vi "New Block UI.vi"(11 "Starting Name":string) -> (2 "Cancelled?":bool, 3 "New Block Config":T1={"Name"="", "Actions"={"Init"=FALSE, "Start"=FALSE, "Run"=TRUE, "Stop"=FALSE, "Close"=FALSE}, "IO Control"=FALSE, "New Project?"=FALSE, "Project"=refnum})   [LabVIEW 2022 SP3, in "FlexBlocks Support.lvlib"]
uses:
  FlexBlocks Support.lvlib
  Action Selections.ctl
  New Block Config.ctl
panel:
  in  "Enable IO Control":bool
  out "Action Diagram":picture
  out "Action Name":string
  out "Info":string
  in  "Actions":T2
  in  "Project Select":string(combo)
  in  "Add To Project":bool
  in  "Cancel":bool
  in  "OK":bool
  # "Enter the name of the new Worker to create:"
  # "Mouseover actions for descriptions."
  # "Unselected actions can later be added to workers by adding the specific case selection back in the Work.vi"
  # "Other Options"
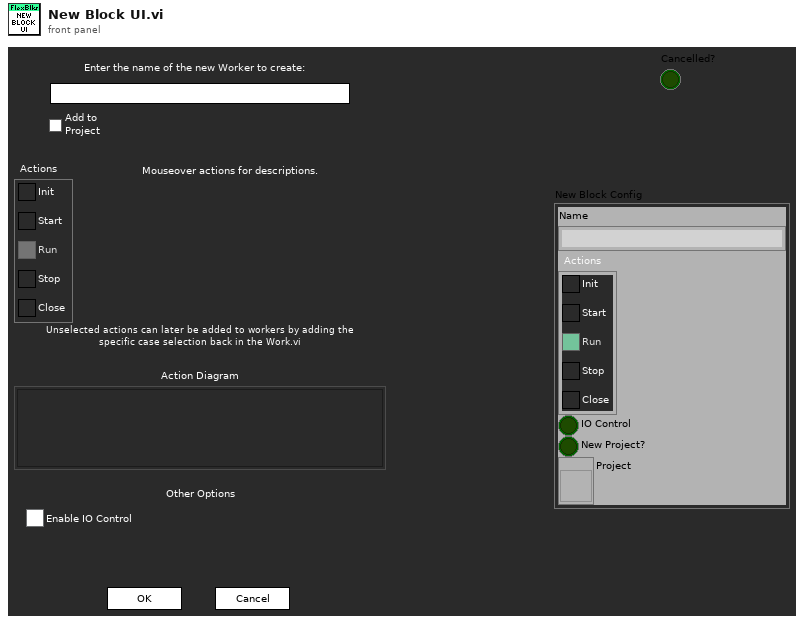
[diagram p1: front panel]
types:
  T1 = typedef "FlexBlocks Support.lvlib/New Block Config.ctl" = cluster{"Name":string, "Actions":T2, "IO Control":bool, "New Project?":bool, "Project":refnum<vi>}
  T2 = typedef "FlexBlocks Support.lvlib/Action Selections.ctl" = cluster{"Init":bool, "Start":bool, "Run":bool, "Stop":bool, "Close":bool}
  T3 = cluster{"Init":bool, "Start":bool, "Run":bool, "Stop":bool, "Close":bool}
  T4 = typedef "FlexBlocks Support.lvlib/Paths.ctl" = cluster{"FlexBlocks":path, "Workers Root":path, "Specialized Editors":path, "Worker Template":path, "SM Template":path, "Read Control Value Vim":path, "Write Indicator Value Vim":path, "XNode":path}
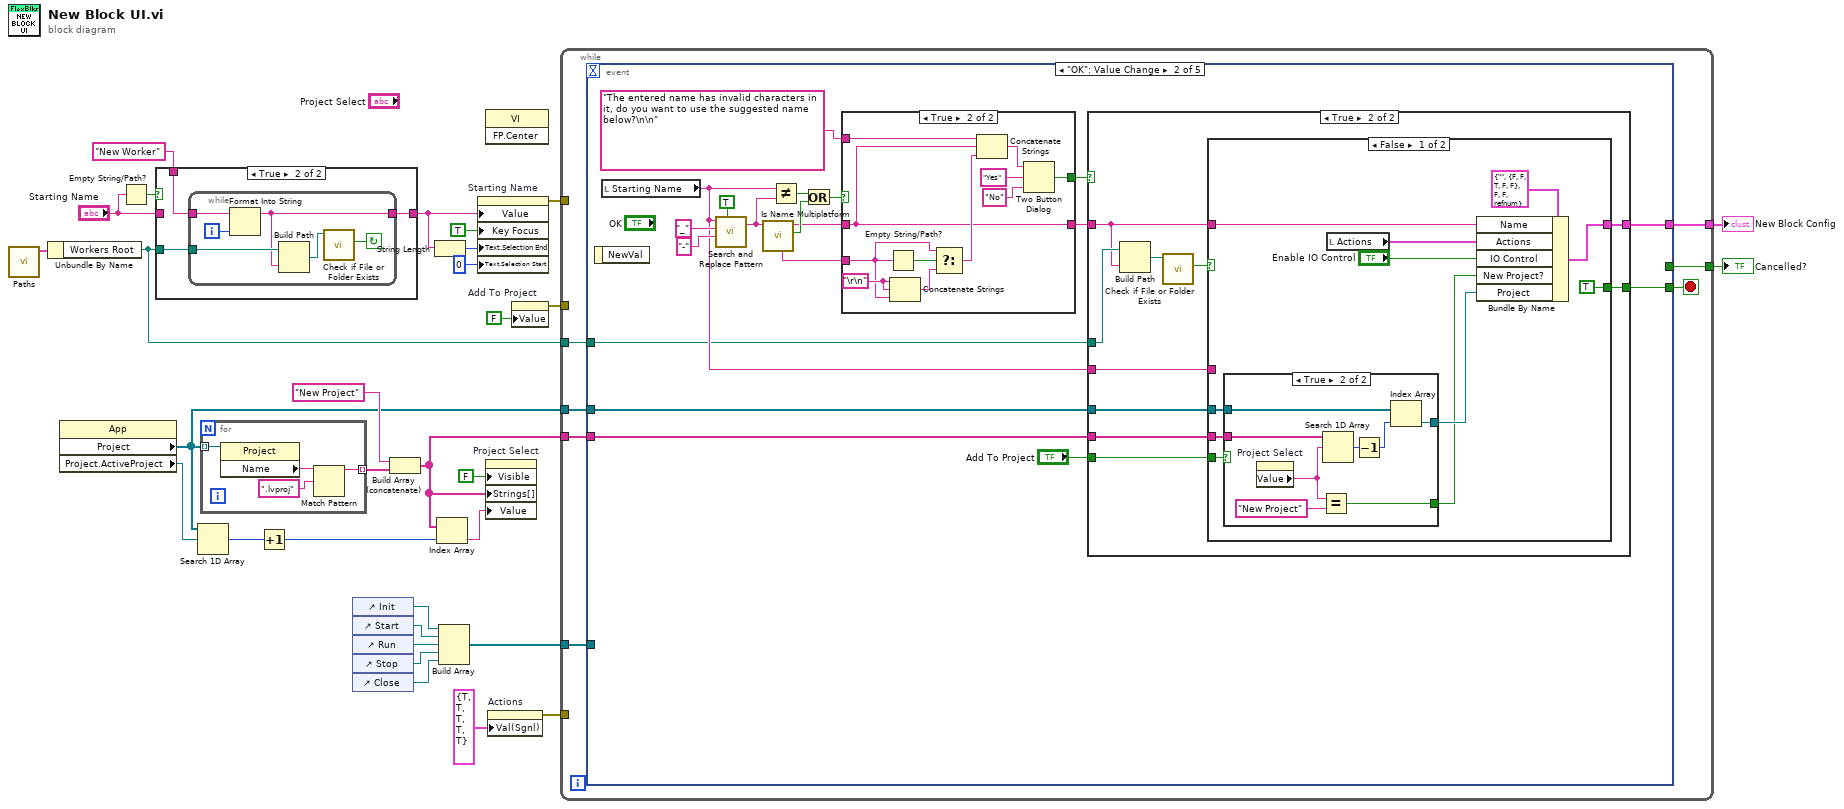
[diagram p0: block diagram]
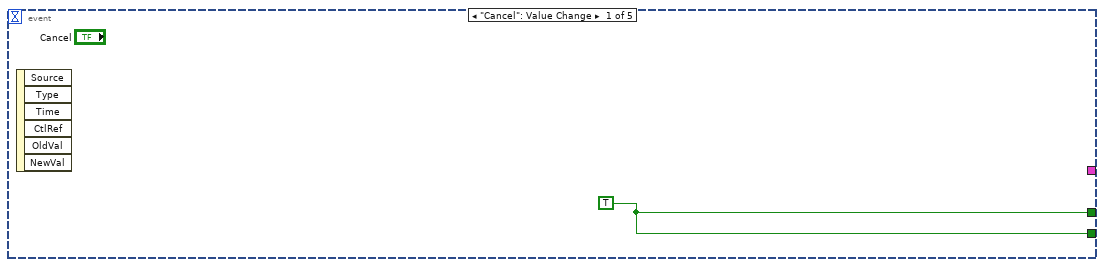
[diagram p2: hidden frame]
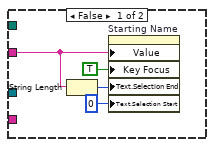
[diagram p3: hidden frame]
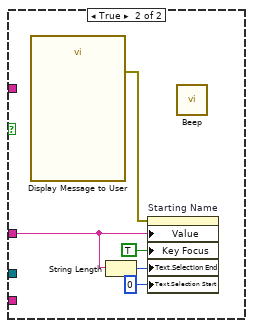
[diagram p5: hidden frame]
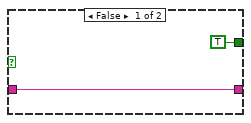
[diagram p6: hidden frame]
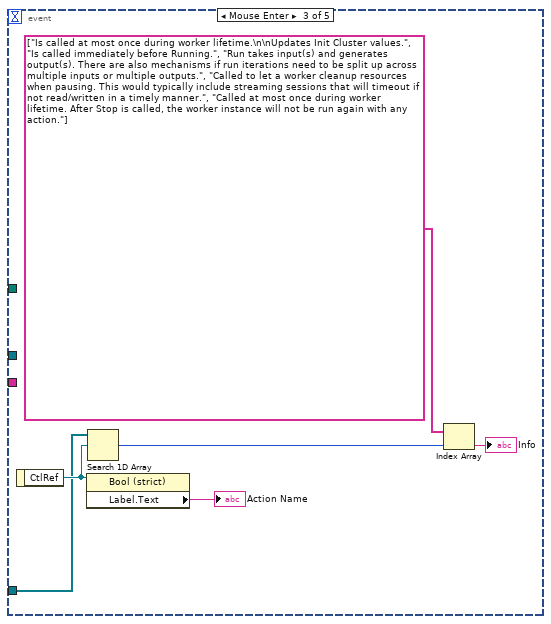
[diagram p7: hidden frame]
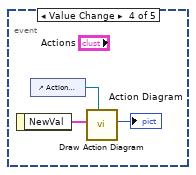
[diagram p8: hidden frame]
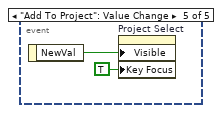
[diagram p9: hidden frame]
diagram:
  n1 = call "Paths.vi"() -> ("Paths"=w16:T4)  [unwired: 11 in]
  n2 = Unbundle By Name(w16) -> ("Workers Root"=w10:path)
  n3 = property class="App"() -> ("Project"=w13:refnum<vi>[], "Project.ActiveProject"=w22:refnum<vi>)  [unwired: 2 in, 2 out]
  n4 = Empty String/Path?(string/path="Starting Name") -> (empty?=w29:bool)
  n5 = case shown="True" w29 {
    tunnel: "Starting Name" -> [w32 _]
    tunnel: w10 -> [_ w35]
    tunnel: [w32 w34] -> w25
    tunnel: "New Worker" -> [_ w33]
    frame False {
    }
    frame True {
      n6 = while {
        tunnel: w35 -> [w40]
        tunnel: [w37] -> w34
        tunnel: w33 -> [w36]
        i -> [w41]
        stop <- w38 continue-if-true
        n7 = Format Into String(initial string=w36, w41) -> (resulting string=w37:string)  [unwired: 2 in, 1 out]
        n8 = Build Path(base path=w40, name or relative path=w37) -> (appended path=w39:path)
        n9 = call <vilib>:"Check if File or Folder Exists.vi"("path"=w39) -> ("file or folder exists?"=w38:bool)  [unwired: 8 in, 2 out]
      }
    }
  }
  n10 = Search 1D Array(1D array=w13, element=w22) -> (index of element=w21:i32)  [unwired: 1 in]
  n11 = for {
    tunnel: w13 -> [w45] mode=indexing
    tunnel: [w42] -> w19 mode=indexing
    n12 = property class="Project"(reference=w45) -> ("Name"=w44:string)  [unwired: 1 in, 2 out]
    n13 = Match Pattern(string=w44, regular expression=".lvproj") -> (before substring=w42:string)  [unwired: 1 in, 3 out]
  }
  n14 = Increment(x=w21) -> (x+1=w17:i32)
  n15 = control-ref of="Init"() -> (w5:refnum<vi>)
  n16 = control-ref of="Start"() -> (w6:refnum<vi>)
  n17 = control-ref of="Run"() -> (w9:refnum<vi>)
  n18 = control-ref of="Stop"() -> (w8:refnum<vi>)
  n19 = control-ref of="Close"() -> (w7:refnum<vi>)
  n20 = Build Array (concatenate)("New Project", w19) -> (w12:string[])
  n21 = String Length(string=w25) -> (length=w27:i32)
  n22 = Index Array(array=w12, index=w17) -> (element=w20:string)
  n23 = Build Array(w5, w6, w9, w8, w7) -> (w4:refnum<vi>[])
  n24 = property on="Starting Name" class="Str"("Value"=w25, "Key Focus"=TRUE, "Text.Selection End"=w27, "Text.Selection Start"=u32 0 ("Text.Selection:Start")) -> (error out=w15:errorcluster)  [unwired: 2 in, 1 out]
  n25 = invoke class="VI" method="FP.Center"() -> ()  [unwired: 3 in, 3 out]
  n26 = property on="Project Select" class="CmbBox"("Visible"=FALSE, "Strings[]"=w12, "Value"=w20) -> ()  [unwired: 2 in, 2 out]
  n27 = property on="Actions" class="Clust (strict)"("Val(Sgnl)"=T3 {"Init"=TRUE, "Start"=TRUE, "Run"=TRUE, "Stop"=TRUE, "Close"=TRUE} ("Value (Signaling)")) -> (error out=w3:errorcluster)  [unwired: 2 in, 1 out]
  n28 = property on="Add To Project" class="Bool (strict)"("Value"=FALSE ("Add To Project")) -> (error out=w14:errorcluster)  [unwired: 2 in, 1 out]
  n29 = while {
    tunnel: w15 -> [_]
    tunnel: w14 -> [_]
    tunnel: w13 -> [w50]
    tunnel: w12 -> [w49]
    tunnel: [w51] -> w11
    tunnel: [w48] -> w1
    tunnel: w10 -> [w47]
    tunnel: w4 -> [w46]
    tunnel: w3 -> [_]
    stop <- w52 stop-if-true
    n30 = event shown="[1] \"OK\": Value Change" {
      selector: _ -> [_ _ _ _ _]
      dyn-events: _ -> [_ _ _ _ _]
      timeout: _ -> [_ _ _ _ _]
      tunnel: [w53 w57 _ _ _] -> w52
      tunnel: [w53 _ _ _ _] -> w51
      tunnel: w50 -> [_ w59 _ _ _]
      tunnel: w49 -> [_ w58 _ _ _]
      tunnel: [_ w56 _ _ _] -> w48
      tunnel: w47 -> [_ w54 _ _ _]
      tunnel: w46 -> [_ _ w127 _ _]
      event "Cancel": Value Change {
        w53 = TRUE
        n31 = event-data() -> ()  [unwired: 1 in, 6 out]
      }
      event "OK": Value Change {
        n32 = event-data() -> ()  [unwired: 1 in, 1 out]
        n33 = local read "Starting Name"() -> (w55:string)
        n34 = call <vilib>:"Search and Replace Pattern.vi"("string"=w55, "regular expression (\"\")"="_" ("regular expression (\"\")"), "replace string (\"\")"="-" ("replace string (\"\")"), "replace all? (F)"=TRUE) -> ("result string"=w66:string)  [unwired: 1 in, 1 out]
        n35 = call <vilib>:"Is Name Multiplatform.vi"("filename"=w66) -> ("filename had conflict"=w71:bool, "suggested filename"=w70:string, "problem description"=w72:string)  [unwired: 6 in, 2 out]
        n36 = Not Equal?(x=w55, y=w66) -> (x != y?=w64:bool)
        n37 = Or(x=w64, y=w71) -> (x .or. y?=w65:bool)
        n38 = case shown="True" w65 {
          tunnel: w72 -> [_ w117]
          tunnel: w70 -> [w112 w113]
          tunnel: "The entered name has invalid characters in it, do you want to use the suggested name below?\n\n" -> [_ w121]
          tunnel: [TRUE ("T button?") w114] -> w61
          tunnel: [w112 w113] -> w62
          frame False {
          }
          frame True {
            w119 = "\r\n"
            n39 = Empty String/Path?(string/path=w117) -> (empty?=w120:bool)
            n40 = Concatenate Strings(w119, w119, w117) -> (w118:string)
            n41 = Select(t=w117, s=w120, f=w118) -> (s? t:f=w116:string)
            n42 = Concatenate Strings(w121, w113, w116) -> (w115:string)
            n43 = Two Button Dialog(message=w115, 1:"No" ("F button name (\"Cancel\")"), 2:"Yes" ("T button name (\"OK\")")) -> (T button?=w114:bool)
          }
        }
        n44 = case shown="True" w61 {
          tunnel: w62 -> [_ w82]
          tunnel: w54 -> [_ w86]
          tunnel: [_ w83] -> w57
          tunnel: [_ w81] -> w56
          tunnel: w55 -> [w73 w80]
          tunnel: w58 -> [_ w79]
          tunnel: w59 -> [_ w78]
          tunnel: "Add To Project" -> [_ w77]
          frame False {
            n45 = String Length(string=w73) -> (length=w76:i32)
            n46 = property on="Starting Name" class="Str"("Value"=w73, "Key Focus"=TRUE, "Text.Selection End"=w76, "Text.Selection Start"=u32 0 ("Text.Selection:Start")) -> ()  [unwired: 2 in, 2 out]
          }
          frame True {
            n47 = Build Path(base path=w86, name or relative path=w82) -> (appended path=w85:path)
            n48 = call <vilib>:"Check if File or Folder Exists.vi"("path"=w85) -> ("file or folder exists?"=w84:bool)  [unwired: 8 in, 2 out]
            n49 = case shown="False" w84 {
              tunnel: [TRUE _] -> w83
              tunnel: w82 -> [w92 _]
              tunnel: [w90 _] -> w81
              tunnel: w80 -> [_ w106]
              tunnel: w79 -> [w95 _]
              tunnel: w78 -> [w94 _]
              tunnel: w77 -> [w96 _]
              frame False {
                n50 = case shown="True" w96 {
                  tunnel: w95 -> [_ w105]
                  tunnel: w94 -> [_ w104]
                  tunnel: [_ w102] -> w88
                  tunnel: [_ w99] -> w87
                  frame False {
                  }
                  frame True {
                    n51 = property on="Project Select" class="CmbBox"() -> ("Value"=w101:string)  [unwired: 2 in, 2 out]
                    n52 = Equal?(x=w101, y="New Project") -> (x = y?=w99:bool)
                    n53 = Search 1D Array(1D array=w105, element=w101) -> (index of element=w103:i32)  [unwired: 1 in]
                    n54 = Decrement(x=w103) -> (x-1=w98:i32)
                    n55 = Index Array(array=w104, index=w98) -> (element=w102:refnum<vi>)
                  }
                }
                n56 = local read "Actions"() -> (w91:T2)
                n57 = Bundle By Name(cluster=T1 {"Name"="", "Actions"={"Init"=FALSE, "Start"=FALSE, "Run"=TRUE, "Stop"=FALSE, "Close"=FALSE}, "IO Control"=FALSE, "New Project?"=FALSE, "Project"=refnum} ("New Block Config"), "Name"=w92, "Actions"=w91, "IO Control"="Enable IO Control", "New Project?"=w87, "Project"=w88) -> (w90:T1)
              }
              frame True {
                n58 = call "Display Message to User"() -> ("error out"=w107:errorcluster)  [unwired: 10 in, 1 out]
                n59 = String Length(string=w106) -> (length=w109:i32)
                n60 = property on="Starting Name" class="Str"(error in=w107, "Value"=w106, "Key Focus"=TRUE, "Text.Selection End"=w109, "Text.Selection Start"=u32 0 ("Text.Selection:Start")) -> ()  [unwired: 1 in, 2 out]
                n61 = call <vilib>:"Beep.vi"() -> ()  [unwired: 12 in]
              }
            }
          }
        }
      }
      event Mouse Enter {
        n62 = event-data() -> ("CtlRef"=w128:refnum<vi>)  [unwired: 1 in]
        n63 = property class="Bool (strict)"(reference=w128) -> ("Label.Text"=→"Action Name":string)  [unwired: 1 in, 2 out]
        n64 = Search 1D Array(1D array=w127, element=w128) -> (index of element=w126:i32)  [unwired: 1 in]
        n65 = Index Array(array=string[] ["Is called at most once during worker lifetime.\n\nUpdates Init Cluster values.", "Is called immediately before Running.", "Run takes input(s) and generates output(s). There are also mechanisms if run iterations need to be split up across multiple inputs or multiple outputs.", "Called to let a worker cleanup resources when pausing. This would typically include streaming sessions that will timeout if not read/written in a timely manner.", "Called at most once during worker lifetime. After Stop is called, the worker instance will not be run again with any action."], index=w126) -> (element=→"Info":string)
      }
      event Value Change {
        n66 = event-data() -> ("NewVal"=w132:T2)  [unwired: 1 in]
        n67 = control-ref of="Action Diagram"() -> (w130:refnum<vi>)
        n68 = call "Draw Action Diagram.vi"("Diagram Ref"=w130, "Actions"=w132) -> ("Action Diagram"=→"Action Diagram":picture)  [unwired: 9 in]
      }
      event "Add To Project": Value Change {
        n69 = event-data() -> ("NewVal"=w133:bool)  [unwired: 1 in]
        n70 = property on="Project Select" class="CmbBox"("Visible"=w133, "Key Focus"=TRUE) -> ()  [unwired: 2 in, 2 out]
      }
    }
  }
  "Cancelled?" <- w11
  "New Block Config" <- w1
